vi "Create Shared Resources.vi"(8 "error in":errorcluster, 10 "custom device ref":T8=18446744073709551615 format="%.0x", 11 "Shared Resources Factory in":refnum<class "Shared Resources Factory.lvclass">) -> (0 "error out":errorcluster, 2 "shared resources":refnum<class "Shared Resources.lvclass">, 3 "Shared Resources Factory out":refnum<class "Shared Resources Factory.lvclass">)   [LabVIEW 2020, in "AIM MIL-STD-1553 Engine.lvlib" / "Implementation.lvlib" / "Shared Resources Factory.lvclass"]
uses:
  Shared Resources Factory.lvclass
  Shared Resources/Shared Resources.lvclass
  Scripting/AIM MIL-STD-1553 Scripting.lvlib
  Shared/Data Word Format.ctl
  Custom Device/Logging Configuration.ctl
  Custom Device/Custom Device.lvlib
  C:/Dev/GitHub/niveristand-aim-milStd1553-custom-device/Source/Custom Device Support/Engine/Implementation/Shared Resources/Shared Resources.lvclass
  C:/Dev/GitHub/niveristand-aim-milStd1553-custom-device/Source/Custom Device Support/Engine/Interfaces/Shared Resources/Shared Resources.lvclass
  <vilib>/NI VeriStand/Custom Device API/Custom Device Item Ref.ctl
  <vilib>/NI VeriStand/Custom Device API/Custom Device API.lvlib
  Interfaces/Shared Resources/Shared Resources.lvclass
  Custom Device/Major Frame Configuration.ctl
  Custom Device/Minor Frame Configuration.ctl
  Custom Device/Message Configuration.ctl
  Custom Device/Bus Controller Configuration.ctl
  Shared/Direction.ctl
  Custom Device/Remote Terminal Configuration.ctl
  Custom Device/1553 Configuration.ctl
panel:
  out "1553 Configuration":T1
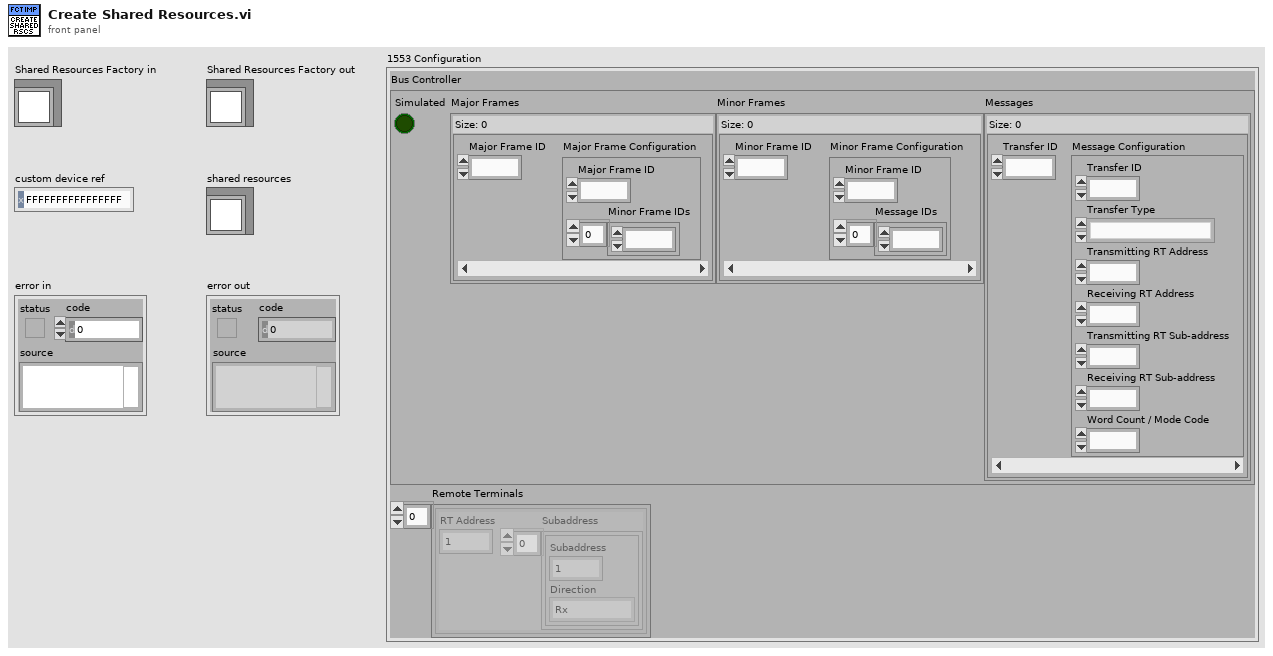
[diagram p1: front panel]
types:
  T1 = typedef "AIM MIL-STD-1553 Engine.lvlib/Custom Device.lvlib/1553 Configuration.ctl" = cluster{"Bus Controller":T2, "Remote Terminals":T6[]}
  T2 = typedef "AIM MIL-STD-1553 Engine.lvlib/Custom Device.lvlib/Bus Controller Configuration.ctl" = cluster{"Simulated":bool, "Major Frames":map{u8, T3}, "Minor Frames":map{u8, T4}, "Messages":map{u16, T5}}
  T3 = typedef "AIM MIL-STD-1553 Engine.lvlib/Custom Device.lvlib/Major Frame Configuration.ctl" = cluster{"Major Frame ID":u8, "Minor Frame IDs":u8[]}
  T4 = typedef "AIM MIL-STD-1553 Engine.lvlib/Custom Device.lvlib/Minor Frame Configuration.ctl" = cluster{"Minor Frame ID":u8, "Message IDs":u16[]}
  T5 = typedef "AIM MIL-STD-1553 Engine.lvlib/Custom Device.lvlib/Message Configuration.ctl" = cluster{"Transfer ID":u16, "Transfer Type":enum16{"BC to RT transfer", "RT to BC transfer", "RT to RT transfer"}, "Transmitting RT Address":u8, "Receiving RT Address":u8, "Transmitting RT Sub-address":u8, "Receiving RT Sub-address":u8, "Word Count / Mode Code":u8}
  T6 = typedef "AIM MIL-STD-1553 Engine.lvlib/Custom Device.lvlib/Remote Terminal Configuration.ctl" = cluster{"RT Address":u8, "Subaddress":cluster{"Subaddress":u8, "Direction":T7}[]}
  T7 = typedef "Direction.ctl" = enum16{"Rx", "Tx"}
  T8 = typedef "Custom Device API.lvlib/Custom Device Item Ref.ctl" = u64
  T9 = typedef "AIM MIL-STD-1553 Engine.lvlib/Custom Device.lvlib/Logging Configuration.ctl" = cluster{"configured":bool, "directory":string, "file name":string, "timestamp file name":bool, "data word format":T10}
  T10 = typedef "Data Word Format.ctl" = string
  T11 = typedef "Device Parameters.ctl" = cluster{"initialization method":T12, "card number":i32, "PXI slot number":i32, "core number":i32}
  T12 = typedef "Initialization Method.ctl" = enum16{"PXI Slot Number", "Card Number"}
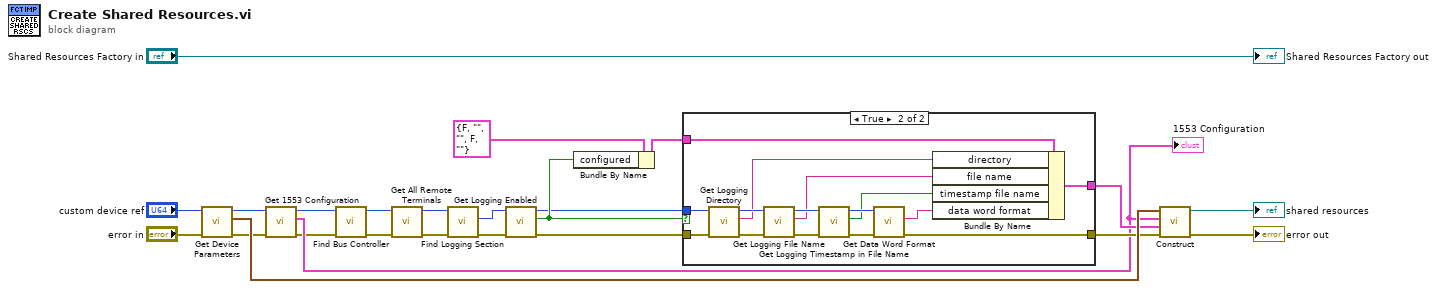
[diagram p0: block diagram]
diagram:
  n1 = call "Get Device Parameters.vi"("error in"="error in", "Ballard MIL-STD 1553 custom device in"="custom device ref") -> ("error out"=w3:errorcluster, "device parameters"=w20:T11, "Ballard MIL-STD 1553 custom device out"=w4:T8)  [unwired: 7 in]
  n2 = call "Get 1553 Configuration.vi"("error in"=w3, "custom device in"=w4) -> ("error out"=w2:errorcluster, "1553 Configuration"=w5:T1, "custom device out"=w1:T8)  [unwired: 7 in]
  "1553 Configuration" <- w5
  n3 = call "Find Bus Controller.vi"("error in"=w2, "port in"=w1) -> ("error out"=w6:errorcluster, "port out"=w7:T8)  [unwired: 6 in, 2 out]
  n4 = call "Get All Remote Terminals.vi"("error in"=w6, "port in"=w7) -> ("error out"=w8:errorcluster, "port out"=w9:T8)  [unwired: 7 in, 1 out]
  n5 = call "Find Logging Section.vi"("error in"=w8, "Ballard MIL-STD 1553 custom device in"=w9) -> ("error out"=w19:errorcluster, "logging"=w18:T8)  [unwired: 7 in, 1 out]
  n6 = call "Get Logging Enabled.vi"("error in"=w19, "logging in"=w18) -> ("error out"=w17:errorcluster, "logging enabled"=w15:bool, "logging out"=w14:T8)  [unwired: 7 in]
  n7 = Bundle By Name(cluster=T9 {"configured"=FALSE, "directory"="", "file name"="", "timestamp file name"=FALSE, "data word format"=""} ("logging configuration"), "configured"=w15) -> (w13:T9)
  n8 = case shown="True" w15 {
    tunnel: w17 -> [w26 w41]
    tunnel: w14 -> [_ w40]
    tunnel: w13 -> [w25 w36]
    tunnel: [w26 w28] -> w12
    tunnel: [w25 w27] -> w11
    frame False {
    }
    frame True {
      n9 = call "Get Logging Directory.vi"("error in"=w41, "logging in"=w40) -> ("error out"=w39:errorcluster, "directory"=w32:string, "logging out"=w35:T8)  [unwired: 7 in]
      n10 = call "Get Logging File Name.vi"("error in"=w39, "logging in"=w35) -> ("error out"=w38:errorcluster, "file name"=w31:string, "logging out"=w34:T8)  [unwired: 7 in]
      n11 = call "Get Logging Timestamp in File Name.vi"("error in"=w38, "logging in"=w34) -> ("error out"=w37:errorcluster, "timestamp in file name"=w30:bool, "logging out"=w33:T8)  [unwired: 7 in]
      n12 = call "Get Data Word Format.vi"("error in"=w37, "logging in"=w33) -> ("error out"=w28:errorcluster, "data word format"=w29:T10)  [unwired: 7 in, 1 out]
      n13 = Bundle By Name(cluster=w36, "directory"=w32, "file name"=w31, "timestamp file name"=w30, "data word format"=w29) -> (w27:T9)
    }
  }
  n14 = call "Construct.vi"("error in"=w12, "logging configuration"=w11, "1553 Configuration"=w5, "device parameters"=w20) -> ("error out"=→"error out":errorcluster, "Ballard 1553 shared resources"=→"shared resources":refnum<class "Shared Resources.lvclass">)  [unwired: 6 in]
  "Shared Resources Factory out" <- "Shared Resources Factory in"
